vi "PXI-Clear Tasks.vi"(0 "AO Tasks":T1[](array[typedef])=[{"Task name"="AO02", "Task"="", "Dual-channel task?"=FALSE, "Regenerate?"=FALSE, "Clear?"=FALSE}], 1 "DI Tasks":T1[](array[typedef]), 2 "DO Tasks":T1[](array[typedef]), 5 "AI Tasks":T1[](array[typedef])=[{"Task name"="AI01", "Task"="", "Dual-channel task?"=FALSE, "Regenerate?"=FALSE, "Clear?"=FALSE}], 7 "Counter Task":T1={"Task name"="Counter", "Task"="", "Dual-channel task?"=FALSE, "Regenerate?"=FALSE, "Clear?"=FALSE}, 11 "error in (no error)":errorcluster, 12 "timeout (sec)":dbl=20.0) -> (15 "error out":errorcluster)   [LabVIEW 2020]
uses:
  Type Defs/Task Struct.ctl
  PXI Globals.vi
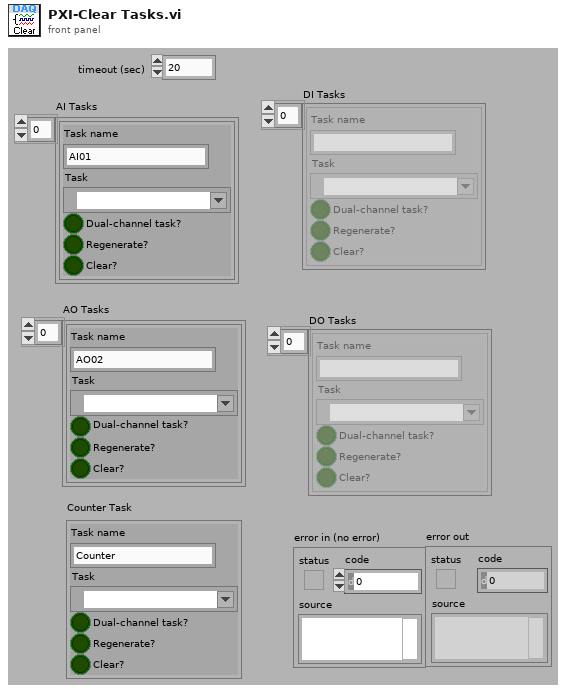
[diagram p1: front panel]
types:
  T1 = typedef "Task Struct.ctl" = cluster{"Task name":string, "Task":refnum<k21>, "Dual-channel task?":bool, "Regenerate?":bool, "Clear?":bool}
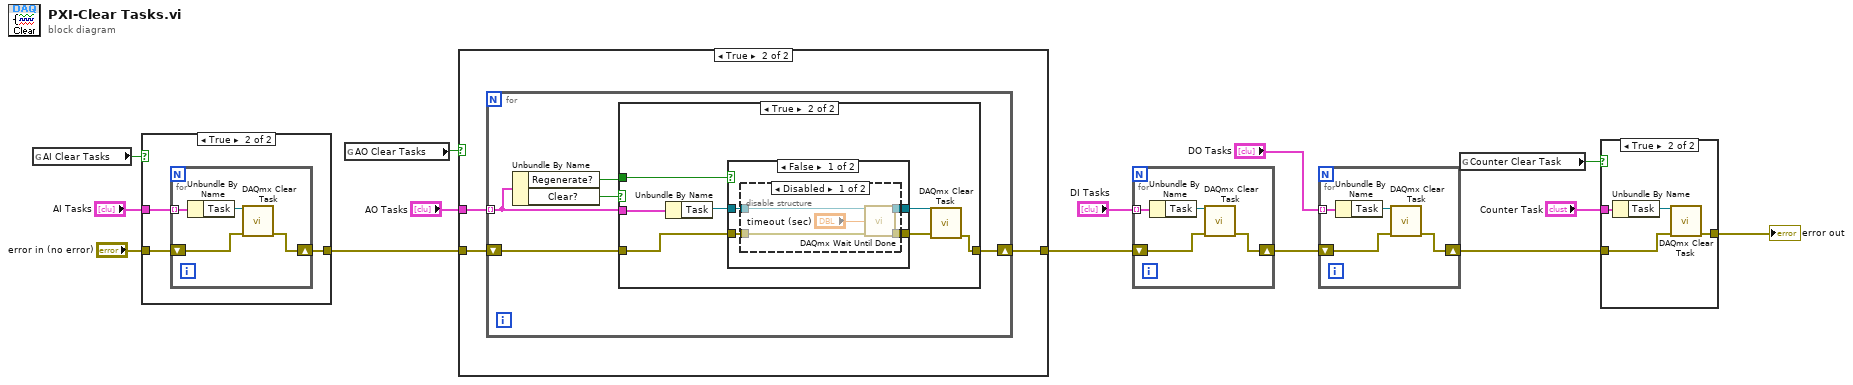
[diagram p0: block diagram]
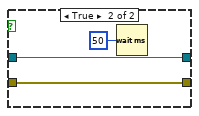
[diagram p6: hidden frame]
diagram:
  n1 = global read "PXI Globals.vi" "AI Clear Tasks"() -> (w11:bool)
  n2 = case shown="True" w11 {
    tunnel: "AI Tasks" -> [_ w18]
    tunnel: "error in (no error)" -> [w15 w17]
    tunnel: [w15 w16] -> w13
    frame False {
    }
    frame True {
      n3 = for {
        tunnel: w18 -> [w22] mode=indexing
        shift-right: [w19] -> w16
        shift-left: w17 -> [w20]
        n4 = Unbundle By Name(w22) -> ("Task"=w21:refnum<k21>)
        n5 = call <vilib>:"DAQmx Clear Task.vi"("task in"=w21, "error in"=w20) -> ("error out"=w19:errorcluster)  [unwired: 13 in]
      }
    }
  }
  n6 = global read "PXI Globals.vi" "AO Clear Tasks"() -> (w10:bool)
  n7 = case shown="True" w10 {
    tunnel: "AO Tasks" -> [_ w26]
    tunnel: [w23 w25] -> w5
    tunnel: w13 -> [w23 w24]
    frame False {
    }
    frame True {
      n8 = for {
        tunnel: w26 -> [w29] mode=indexing
        shift-right: [w30] -> w25
        shift-left: w24 -> [w31]
        n9 = Unbundle By Name(w29) -> ("Regenerate?"=w28:bool, "Clear?"=w27:bool)
        n10 = case shown="True" w27 {
          tunnel: w29 -> [_ w39]
          tunnel: w31 -> [w32 w36]
          tunnel: [w32 w38] -> w30
          tunnel: w28 -> [_ w33]
          frame False {
          }
          frame True {
            n11 = Unbundle By Name(w39) -> ("Task"=w37:refnum<k21>)
            n12 = case shown="False" w33 {
              tunnel: w37 -> [w43 w53]
              tunnel: w36 -> [w42 w52]
              tunnel: [w41 w52] -> w35
              tunnel: [w40 w53] -> w34
              frame False {
                n13 = disable-structure shown="Disabled" {
                  disable-tunnel: w43 -> [w48 w50]
                  disable-tunnel: w42 -> [w47 w49]
                  disable-tunnel: [w46 w49] -> w41
                  disable-tunnel: [w45 w50] -> w40
                  frame Disabled {
                    n14 = call <vilib>:"DAQmx Wait Until Done.vi"("task/channels in"=w48, "timeout (sec)"="timeout (sec)", "error in"=w47) -> ("task out"=w45:refnum<k21>, "error out"=w46:errorcluster)  [unwired: 11 in]
                  }
                  frame Enabled {
                  }
                }
              }
              frame True {
                n15 = Wait (ms)(milliseconds to wait=u32 50) -> ()  [unwired: 1 out]
              }
            }
            n16 = call <vilib>:"DAQmx Clear Task.vi"("task in"=w34, "error in"=w35) -> ("error out"=w38:errorcluster)  [unwired: 13 in]
          }
        }
      }
    }
  }
  n17 = for {
    tunnel: "DI Tasks" -> [w57] mode=indexing
    shift-right: [w54] -> w3
    shift-left: w5 -> [w55]
    n18 = Unbundle By Name(w57) -> ("Task"=w56:refnum<k21>)
    n19 = call <vilib>:"DAQmx Clear Task.vi"("task in"=w56, "error in"=w55) -> ("error out"=w54:errorcluster)  [unwired: 13 in]
  }
  n20 = for {
    tunnel: "DO Tasks" -> [w61] mode=indexing
    shift-right: [w58] -> w2
    shift-left: w3 -> [w59]
    n21 = Unbundle By Name(w61) -> ("Task"=w60:refnum<k21>)
    n22 = call <vilib>:"DAQmx Clear Task.vi"("task in"=w60, "error in"=w59) -> ("error out"=w58:errorcluster)  [unwired: 13 in]
  }
  n23 = global read "PXI Globals.vi" "Counter Clear Task"() -> (w9:bool)
  n24 = case shown="True" w9 {
    tunnel: w2 -> [w62 w66]
    tunnel: "Counter Task" -> [_ w64]
    tunnel: [w62 w63] -> w14
    frame False {
    }
    frame True {
      n25 = Unbundle By Name(w64) -> ("Task"=w65:refnum<k21>)
      n26 = call <vilib>:"DAQmx Clear Task.vi"("task in"=w65, "error in"=w66) -> ("error out"=w63:errorcluster)  [unwired: 13 in]
    }
  }
  "error out" <- w14
